vi "Vector_arrow.vi"(10 "vector":cluster{"length":dbl, "angle":dbl, "sense":bool}, 11 "tip":cluster{dbl, dbl}) -> (3 "(x,y)":cluster{dbl, dbl}[](array[cluster]))   [LabVIEW 2024]
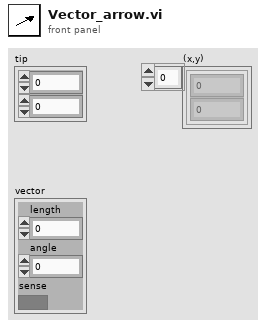
[diagram p1: front panel]
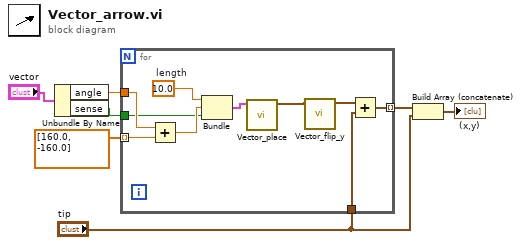
[diagram p0: block diagram]
diagram:
  n1 = Unbundle By Name("vector") -> ("angle"=w3:dbl, "sense"=w1:bool)
  n2 = for {
    tunnel: "tip" -> [w11]
    tunnel: dbl[] [160.0, -160.0] -> [w14] mode=indexing
    tunnel: [w13] -> w5 mode=indexing
    tunnel: w3 -> [w12]
    tunnel: w1 -> [w8]
    w15 = 10.0  # length
    n3 = Add(x=w12, y=w14) -> (x+y=w17:dbl)
    n4 = Bundle("length"=w15, w17, "sense"=w8) -> (w16:cluster{"length":dbl, dbl, "sense":bool})  [unwired: 1 in]
    n5 = call "Vector_place.vi"("vector"=w16) -> ("x,y"=w10:cluster{dbl, dbl})  [unwired: 10 in]
    n6 = call "Vector_flip_y.vi"("x,y"=w10) -> ("x,-y"=w9:cluster{"X ":i16, "Y ":i16})  [unwired: 10 in]
    n7 = Add(x=w9, y=w11) -> (x+y=w13:cluster{dbl, dbl})
  }
  n8 = Build Array (concatenate)(w5, "tip") -> (→"(x,y)":cluster{dbl, dbl}[])
